vi "WriteJump.vi"(5 "Teleop Local Data In":T1 {"Vision"."Theta_Y" format="%.1f"; "Vision"."Theta_X" format="%.1f"; "Potentio" format="%.1f"; "Drive_Enc_R" format="%.1f"; "Drive_Enc_L" format="%.1f"; "Gyro_Angle" format="%.1f"; "Encoder_Lift" format="%.1f"; "Motor_Lift" format="%.3f"; "Motor_Intake" format="%.3f"; "Drive_Twist" format="%.3f"; "Drive_Forward" format="%.3f"}, 9 "error in":errorcluster) -> (6 "Teleop Local Data Out":T1 {"Vision"."Theta_Y" format="%.1f"; "Vision"."Theta_X" format="%.1f"; "Potentio" format="%.1f"; "Drive_Enc_R" format="%.1f"; "Drive_Enc_L" format="%.1f"; "Gyro_Angle" format="%.1f"; "Encoder_Lift" format="%.1f"; "Motor_Lift" format="%.3f"; "Motor_Intake" format="%.3f"; "Drive_Twist" format="%.3f"; "Drive_Forward" format="%.3f"}, 10 "error out":errorcluster)   [LabVIEW 2018]
uses:
  Typedefs/typedef_cluster_TeleOp_Local_Data.ctl
  Typedefs/typedef_cluster_Joystick.ctl
  Typedefs/typedef_cluster_Vision.ctl
  Typedefs/typedef_enum_refnums.ctl
  <vilib>/Rock Robotics/WPI/Solenoid/WPI_SolenoidValue.ctl
  <vilib>/Rock Robotics/WPI/Solenoid/WPI_SolenoidSetEnum.vi
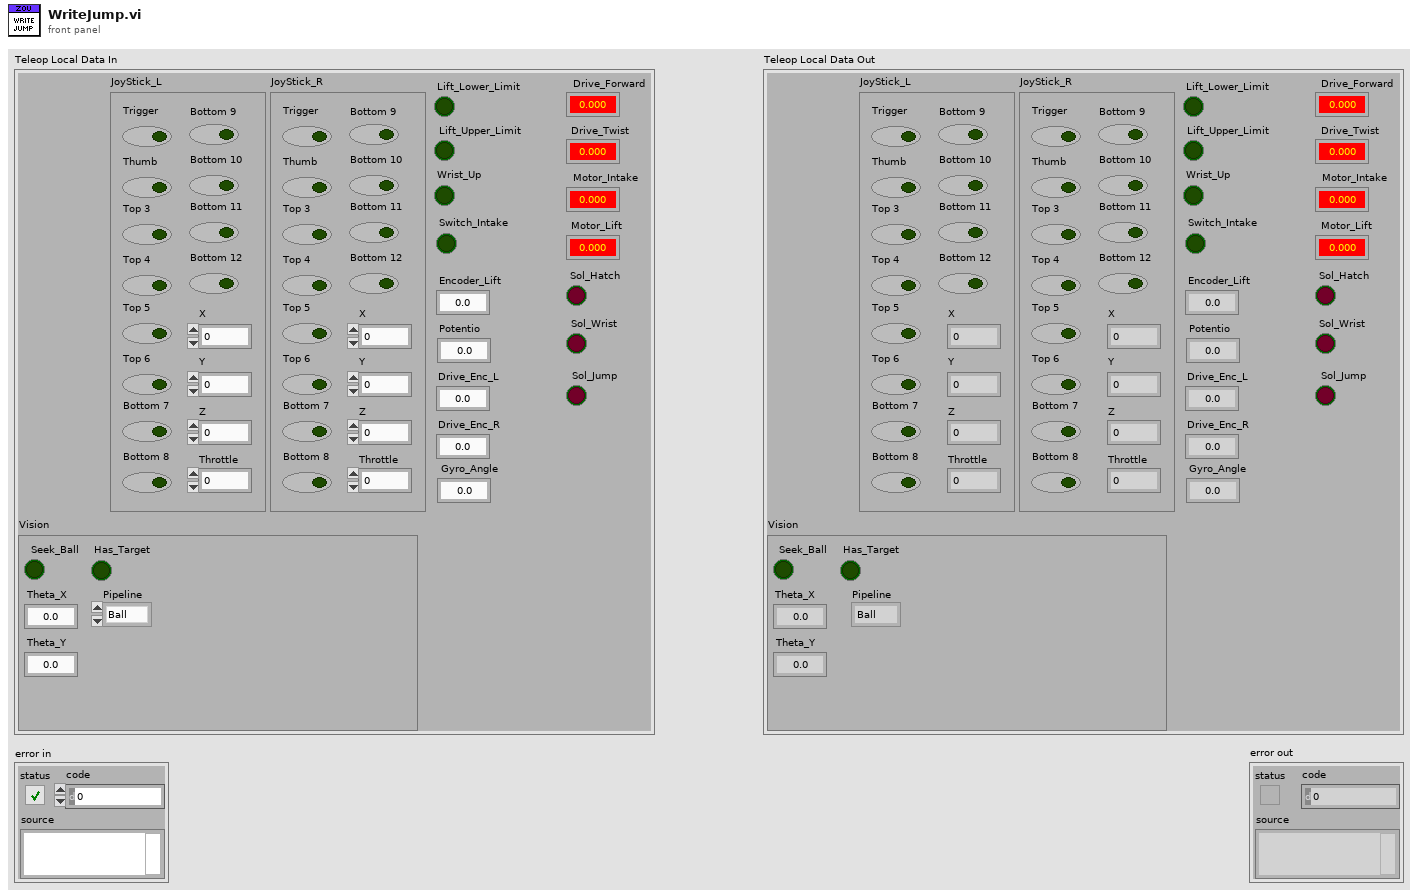
[diagram p1: front panel]
types:
  T1 = typedef "typedef_cluster_TeleOp_Local_Data.ctl" = cluster{"Lift_Lower_Limit":bool, "Wrist_Up":bool, "Switch_Intake":bool, "Encoder_Lift":dbl, "Sol_Wrist":bool, "Motor_Intake":dbl, "Motor_Lift":dbl, "Drive_Forward":dbl, "Drive_Twist":dbl, "Sol_Hatch":bool, "Gyro_Angle":dbl, "Drive_Enc_L":dbl, "Drive_Enc_R":dbl, "JoyStick_L":T2, "JoyStick_R":T2, "Potentio":dbl, "Vision":T3, "Lift_Upper_Limit":bool, "Sol_Jump":bool}
  T2 = typedef "typedef_cluster_Joystick.ctl" = cluster{"X":dbl, "Y":dbl, "Z":dbl, "Throttle":dbl, "Trigger":bool, "Thumb":bool, "Top 3":bool, "Top 4":bool, "Top 5":bool, "Top 6":bool, "Bottom 7":bool, "Bottom 8":bool, "Bottom 9":bool, "Bottom 10":bool, "Bottom 11":bool, "Bottom 12":bool}
  T3 = typedef "typedef_cluster_Vision.ctl" = cluster{"Theta_X":dbl, "Theta_Y":dbl, "Has_Target":bool, "Seek_Ball":bool, "Pipeline":enum16{"Ball", "Dual_Target", "Single_Target"}}
  T4 = typedef "WPI_SolenoidValue.ctl" = enum16{"Off", "On", "Forward", "Reverse"}
  T5 = typedef "typedef_enum_refnums.ctl" = enum16{"Joy_L", "Joy_R", "Drive_Motors", "Intake_Motor", "Wrist_Solenoid", "Hatch_Solenoid", "Compressor", "Lift_Motor", "Lift_Motor_2", "Gyro", "Drive_Enc_L", "Drive_Enc_R", "Lift_Lower_Limit", "Lift_Upper_Limit", "Ball_Switch", "Jump_Solenoid"}
  T6 = typedef "WPI_SolenoidDevRef.ctl" = cluster{"DevStatus":errorcluster, "Pneumatics Control Module":u8, "Forward Solenoid Channel":T7, "Reverse Solenoid Channel":T7}
  T7 = typedef "WPI_SolenoidChannel.ctl" = enum8{"Solenoid 0", "Solenoid 1", "Solenoid 2", "Solenoid 3", "Solenoid 4", "Solenoid 5", "Solenoid 6", "Solenoid 7", "Invalid"}
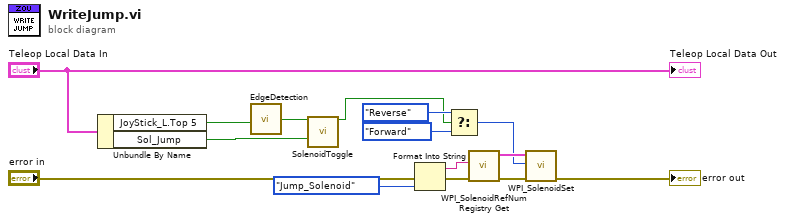
[diagram p0: block diagram]
diagram:
  n1 = Unbundle By Name("Teleop Local Data In") -> ("JoyStick_L.Top 5"=w5:bool, "Sol_Jump"=w1:bool)
  n2 = call "EdgeDetection.vi"("Boolean"=w5) -> ("Boolean 2"=w7:bool)  [unwired: 14 in]
  n3 = call "SolenoidToggle.vi"("Button Press"=w7, "x"=w1) -> ("Boolean"=w6:bool)  [unwired: 13 in]
  n4 = Format Into String(error in="error in", typedef_enum_refnums."Jump_Solenoid" ("Enum")) -> (resulting string=w12:string, error out=w15:errorcluster)  [unwired: 2 in]
  n5 = Select(t=WPI_SolenoidValue."Reverse" ("Value"), s=w6, f=WPI_SolenoidValue."Forward") -> (s? t:f=w8:T4)
  n6 = call <vilib>:"WPI_SolenoidRefNum Registry Get.vi"("error in (no error)"=w15, "refnum name"=w12) -> ("error out"=w13:errorcluster, "SolenoidDevRef"=w11:T6)  [unwired: 8 in]
  n7 = call-poly <vilib>:"WPI_SolenoidSet.vi"("error in (no error)"=w13, "Value"=w8, "SolenoidDevRef"=w11) -> ("error out"=→"error out":errorcluster)  [unwired: 7 in, 1 out]
  "Teleop Local Data Out" <- "Teleop Local Data In"
